vi "Init Add Run Window.vi"(10 "FPGA Names":string[](array[string])) -> (0 "error out":errorcluster)   [LabVIEW 2020, in "Scheduler.lvlib"]
uses:
  Scheduler.lvlib
  Add RUN Window.vi
  Run Utilities/Run Utilities.lvlib
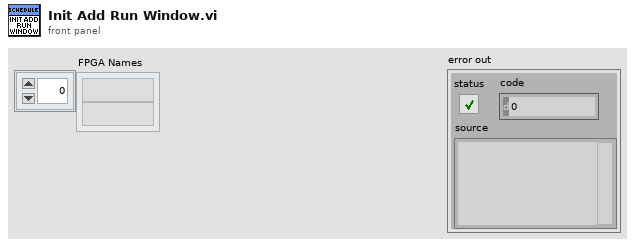
[diagram p1: front panel]
types:
  T1 = cluster{"Parameter Name":string, "Parameter Name":string}
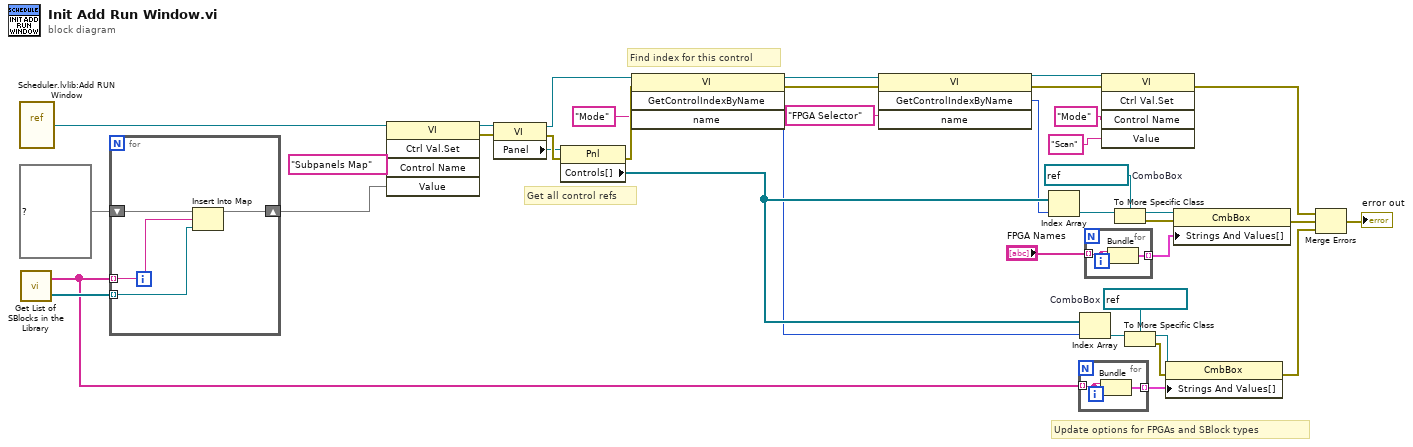
[diagram p0: block diagram]
diagram:
  w9 = refnum<vi> refnum  # ComboBox
  w30 = refnum<vi> refnum  # ComboBox
  # "Update options for FPGAs and SBlock types"
  # "Find index for this control"
  # "Get all control refs"
  n1 = vi-ref "Scheduler.lvlib:Add RUN Window.vi"() -> (w1:refnum<vi>)
  n2 = call "Get List of SBlocks in the Library.vi"() -> ("Subpanel Refs"=w38:refnum<vi>[], "List of Available SBlock Types"=w20:string[])  [unwired: 2 in]
  n3 = for {
    tunnel: w20 -> [w39] mode=indexing
    tunnel: w38 -> [w40] mode=indexing
    shift-right: [w41] -> w36
    shift-left: map{string, refnum<vi>} {} ("Subpanels Map") -> [w42]
    n4 = Insert Into Map(map in=w42, key=w39, value=w40) -> (map out=w41:map{string, refnum<vi>})  [unwired: 2 out]
  }
  n5 = invoke class="VI" method="Ctrl Val.Set"(reference=w1, "Control Name"="Subpanels Map", "Value"=w36) -> (reference out=w23:refnum<vi>, error out=w22:errorcluster)  [unwired: 2 in, 3 out]
  n6 = property class="VI"(reference=w23, error in=w22) -> (reference out=w26:refnum<vi>, error out=w28:errorcluster, "Panel"=w27:refnum<vi>)
  n7 = property class="Pnl"(reference=w27, error in=w28) -> (error out=w25:errorcluster, "Controls[]"=w16:refnum<vi>[])  [unwired: 1 out]
  n8 = invoke class="VI" method="GetControlIndexByName"(reference=w26, error in=w25, "name"="Mode" ("Control Name")) -> (reference out=w19:refnum<vi>, error out=w18:errorcluster, "GetControlIndexByName"=w6:i32)  [unwired: 1 in, 1 out]
  n9 = invoke class="VI" method="GetControlIndexByName"(reference=w19, error in=w18, "name"="FPGA Selector" ("Control Name")) -> (reference out=w14:refnum<vi>, error out=w13:errorcluster, "GetControlIndexByName"=w15:i32)  [unwired: 1 in, 1 out]
  n10 = Index Array(array=w16, index=w15) -> (element=w10:refnum<vi>)
  n11 = for {
    tunnel: w20 -> [w44] mode=indexing
    tunnel: [w43] -> w29 mode=indexing
    n12 = Bundle("Name"=w44, "Name"=w44) -> (w43:cluster{"Name":string, "Name":string})  [unwired: 1 in]
  }
  n13 = Index Array(array=w16, index=w6) -> (element=w24:refnum<vi>)
  n14 = for {
    tunnel: "FPGA Names" -> [w46] mode=indexing
    tunnel: [w45] -> w7 mode=indexing
    n15 = Bundle("Parameter Name"=w46, "Parameter Name"=w46) -> (w45:T1)  [unwired: 1 in]
  }
  n16 = invoke class="VI" method="Ctrl Val.Set"(reference=w14, error in=w13, "Control Name"="Mode", "Value"="Scan" ("Control Name")) -> (error out=w2:errorcluster)  [unwired: 1 in, 4 out]
  n17 = To More Specific Class(target class=w9, reference=w10) -> (specific class reference=w11:refnum<vi>, error out=w12:errorcluster)  [unwired: 1 in]
  n18 = To More Specific Class(target class=w30, reference=w24) -> (specific class reference=w32:refnum<vi>, error out=w31:errorcluster)  [unwired: 1 in]
  n19 = property class="CmbBox"(reference=w32, error in=w31, "Strings And Values[]"=w29) -> (error out=w4:errorcluster)  [unwired: 1 out]
  n20 = property class="CmbBox"(reference=w11, error in=w12, "Strings And Values[]"=w7) -> (error out=w5:errorcluster)  [unwired: 1 out]
  n21 = Merge Errors(w2, w5, w4) -> (→"error out":errorcluster)
